vi "单个流程写入.vi"(7 "添加的路径":path, 8 "error in (no error)":errorcluster caption="错误输入（无错误）", 9 "量程":enum16{"低量程", "高量程"}(ring), 10 "测量模式":enum16{"水样测量", "零点核查", "跨度核查", "标样核查", "加标回收"}(ring), 11 "测量参数":enum16{"COD", "氨氮", "总氮", "总磷"}(ring)) -> (0 "error out":errorcluster caption="错误输出", 3 "步数":i32)   [LabVIEW 2016, in "斯坦道总氮.lvlib"]
panel:
  out "数组 2":u16[][](array[numeric]) format="0x%04x"
  out "大小":i32
  out "交织的数组":u16[](array[numeric]) format="0x%04x"
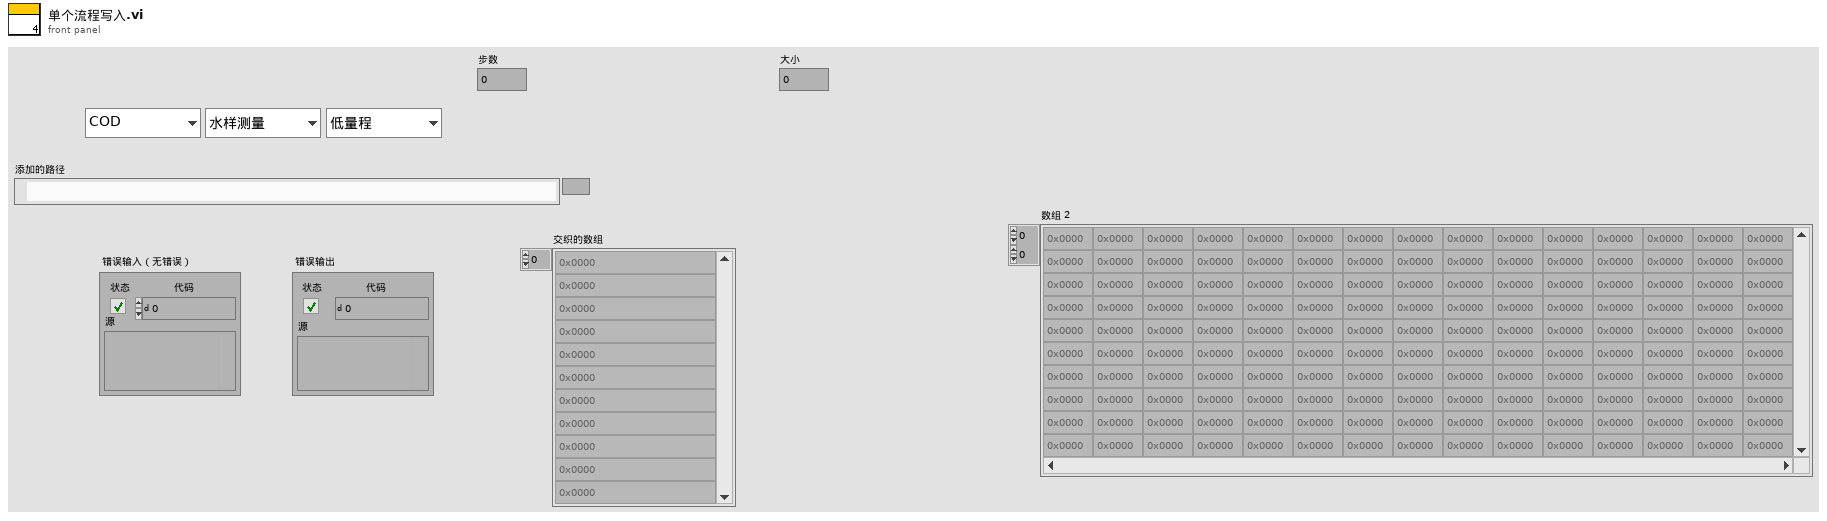
[diagram p1: front panel]
types:
  T1 = cluster{"站号":u16, "starting address":u16, "starting address":u16}
  T2 = cluster{"port":u32, "dac":u8, "adc":u8, "time":u16, "步骤名":string}[]
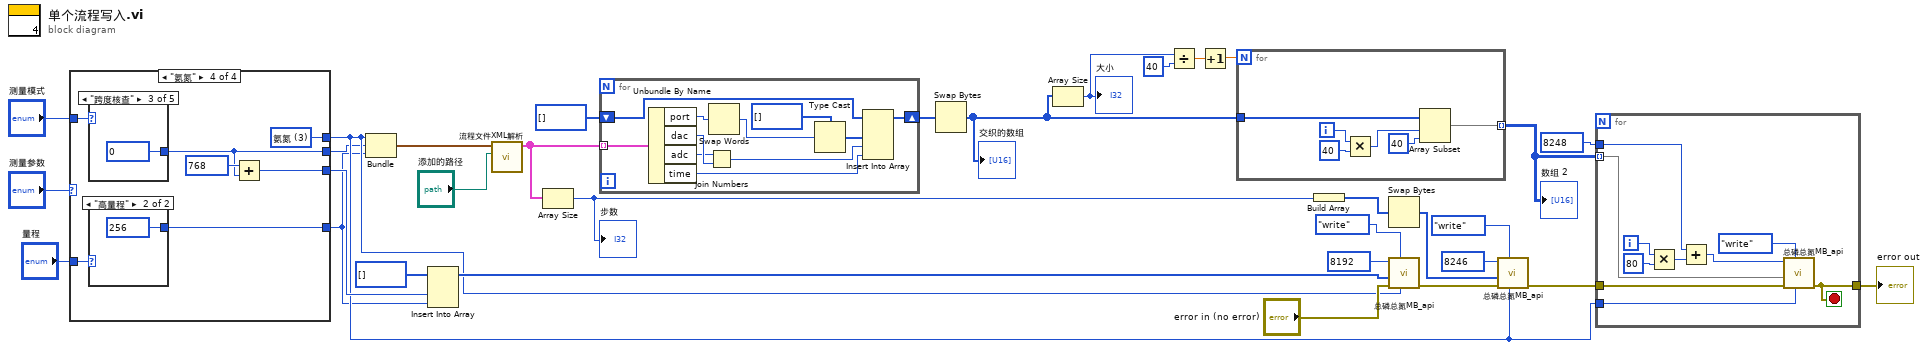
[diagram p0: block diagram]
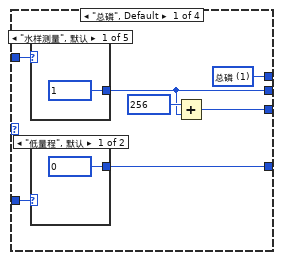
[diagram p2: hidden frame]
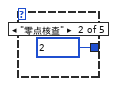
[diagram p3: hidden frame]
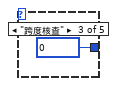
[diagram p4: hidden frame]
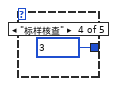
[diagram p5: hidden frame]
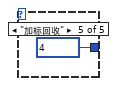
[diagram p6: hidden frame]
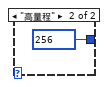
[diagram p7: hidden frame]
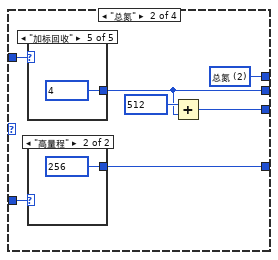
[diagram p8: hidden frame]
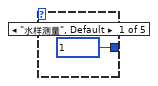
[diagram p9: hidden frame]
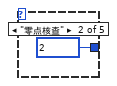
[diagram p10: hidden frame]
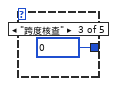
[diagram p11: hidden frame]
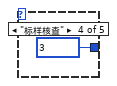
[diagram p12: hidden frame]
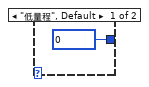
[diagram p13: hidden frame]
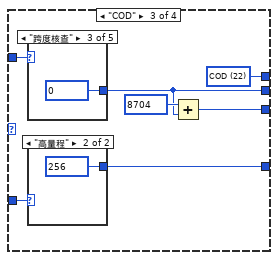
[diagram p14: hidden frame]
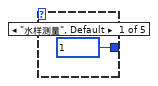
[diagram p15: hidden frame]
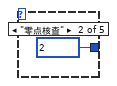
[diagram p16: hidden frame]
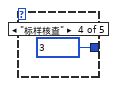
[diagram p17: hidden frame]
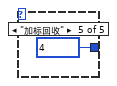
[diagram p18: hidden frame]
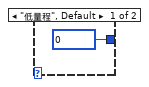
[diagram p19: hidden frame]
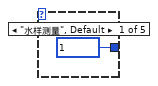
[diagram p20: hidden frame]
diagram:
  n1 = case shown="\"氨氮\"" "测量参数" {
    tunnel: "测量模式" -> [w38 w51 w65 w79]
    tunnel: "量程" -> [w39 w52 w66 w80]
    tunnel: [w34 w53 w67 w81] -> w18
    tunnel: [w35 w48 w62 w76] -> w28
    tunnel: [w37 w50 w64 w78] -> w15
    tunnel: [w33 w47 w61 w75] -> w16
    frame "总磷", Default {
      w34 = u16 1 items=["总磷"=1, "总氮"=2, "氨氮"=3] ("站号")
      n2 = case shown="\"水样测量\", 默认" w38 {
        tunnel: [u16 1 ("starting address") u16 2 ("starting address") u16 0 ("starting address") u16 3 ("starting address") u16 4 ("starting address")] -> w33
        frame "水样测量", Default {
        }
        frame "零点核查" {
        }
        frame "跨度核查" {
        }
        frame "标样核查" {
        }
        frame "加标回收" {
        }
      }
      n3 = case shown="\"低量程\", 默认" w39 {
        tunnel: [u16 0 ("starting address") u16 256 ("starting address")] -> w37
        frame "低量程", Default {
        }
        frame "高量程" {
        }
      }
      n4 = Add(x=u16 256 ("starting address"), y=w33) -> (x+y=w35:u16)
    }
    frame "总氮" {
      w53 = u16 2 items=["总磷"=1, "总氮"=2, "氨氮"=3] ("站号")
      n5 = case shown="\"加标回收\"" w51 {
        tunnel: [u16 1 ("starting address") u16 2 ("starting address") u16 0 ("starting address") u16 3 ("starting address") u16 4 ("starting address")] -> w47
        frame "水样测量", Default {
        }
        frame "零点核查" {
        }
        frame "跨度核查" {
        }
        frame "标样核查" {
        }
        frame "加标回收" {
        }
      }
      n6 = case shown="\"高量程\"" w52 {
        tunnel: [u16 0 ("starting address") u16 256 ("starting address")] -> w50
        frame "低量程", Default {
        }
        frame "高量程" {
        }
      }
      n7 = Add(x=u16 512 ("starting address"), y=w47) -> (x+y=w48:u16)
    }
    frame "COD" {
      w67 = u16 22 items=["总磷"=1, "总氮"=2, "COD"=22] ("站号")
      n8 = case shown="\"跨度核查\"" w65 {
        tunnel: [u16 1 ("starting address") u16 2 ("starting address") u16 0 ("starting address") u16 3 ("starting address") u16 4 ("starting address")] -> w61
        frame "水样测量", Default {
        }
        frame "零点核查" {
        }
        frame "跨度核查" {
        }
        frame "标样核查" {
        }
        frame "加标回收" {
        }
      }
      n9 = case shown="\"高量程\"" w66 {
        tunnel: [u16 0 ("starting address") u16 256 ("starting address")] -> w64
        frame "低量程", Default {
        }
        frame "高量程" {
        }
      }
      n10 = Add(x=u16 8704 ("starting address"), y=w61) -> (x+y=w62:u16)
    }
    frame "氨氮" {
      w81 = u16 3 items=["总磷"=1, "总氮"=2, "氨氮"=3, "COD"=22] ("站号")
      n11 = case shown="\"跨度核查\"" w79 {
        tunnel: [u16 1 ("starting address") u16 2 ("starting address") u16 0 ("starting address") u16 3 ("starting address") u16 4 ("starting address")] -> w75
        frame "水样测量", Default {
        }
        frame "零点核查" {
        }
        frame "跨度核查" {
        }
        frame "标样核查" {
        }
        frame "加标回收" {
        }
      }
      n12 = case shown="\"高量程\"" w80 {
        tunnel: [u16 0 ("starting address") u16 256 ("starting address")] -> w78
        frame "低量程", Default {
        }
        frame "高量程" {
        }
      }
      n13 = Add(x=u16 768 ("starting address"), y=w75) -> (x+y=w76:u16)
    }
  }
  n14 = Bundle("站号"=w18, "starting address"=w16, "starting address"=w15) -> (w14:T1)  [unwired: 1 in]
  n15 = Insert Into Array(array=u16[] [] ("数组"), new element #1=w28, new element #2=w15) -> (w22:u16[])  [unwired: 1 in]
  n16 = call "流程文件XML解析.vi"("添加的路径"="添加的路径", "参数簇"=w14) -> ("数组"=w6:T2)  [unwired: 9 in]
  n17 = Array Size(array=w6) -> (size(s)=w1:i32)
  "步数" <- w1
  n18 = for {
    tunnel: w6 -> [w99] mode=indexing
    shift-right: [w94] -> w11
    shift-left: u16[] [] -> [w92]
    n19 = Unbundle By Name(w99) -> ("port"=w97:u32, "dac"=w90:u8, "adc"=w89:u8, "time"=w95:u16)
    n20 = Join Numbers(hi=w89, lo=w90) -> ((hi.lo)=w96:u16)
    n21 = Swap Words(1:w97) -> (0:w91:u32)
    n22 = Type Cast(type=u16[] [], x=w91) -> (*(type *) &x=w93:u16[])
    n23 = Insert Into Array(array=w92, new element #1=w93, new element #2=w96, new element #3=w95) -> (w94:u16[])  [unwired: 1 in]
  }
  n24 = Swap Bytes(anything=w11) -> (byte swapped=w8:u16[])
  "交织的数组" <- w8
  n25 = Array Size(array=w8) -> (size(s)=w10:i32)
  "大小" <- w10
  n26 = Divide(x=w10, y=40) -> (x/y=w4:dbl)
  n27 = Increment(x=w4) -> (x+1=w3:dbl)
  n28 = for {
    N: w3 -> [_]
    tunnel: w8 -> [w103]
    tunnel: [w100] -> w7 mode=indexing
    i -> [w105]
    n29 = Multiply(x=w105, y=40) -> (x*y=w102:i32)
    n30 = Array Subset(array=w103, index=w102, length=40 ("y")) -> (w100:u16[])
  }
  "数组 2" <- w7
  n31 = Build Array(w1) -> (w5:i32[])
  n32 = Swap Bytes(anything=w5) -> (byte swapped=w2:i32[])
  n33 = call "总磷总氮MB_api.vi"("Slave ID"=w18, "STEP"=enum16{"open", "read", "write", "close"}."write", "Error in"="error in (no error)", "values"=w22, "starting address"=u16 8192) -> ("error out"=w25:errorcluster)  [unwired: 4 in, 2 out]
  n34 = call "总磷总氮MB_api.vi"("Slave ID"=w18, "STEP"=enum16{"open", "read", "write", "close"}."write", "Error in"=w25, "values"=w2, "starting address"=u16 8246) -> ("error out"=w21:errorcluster)  [unwired: 4 in, 2 out]
  n35 = for {
    tunnel: u16 8248 ("starting address") -> [w109]
    tunnel: w21 -> [w115]
    tunnel: [w113] -> w19
    tunnel: w18 -> [w112]
    tunnel: w7 -> [w111] mode=indexing
    i -> [w108]
    stop <- w113 stop-if-true
    n36 = Multiply(x=w108, y=80) -> (x*y=w107:i32)
    n37 = Add(x=w109, y=w107) -> (x+y=w110:i32)
    n38 = call "总磷总氮MB_api.vi"("Slave ID"=w112, "STEP"=enum16{"open", "read", "write", "close"}."write", "Error in"=w115, "values"=w111, "starting address"=w110) -> ("error out"=w113:errorcluster)  [unwired: 4 in, 2 out]
  }
  "error out" <- w19
